vi "user1.vi"() -> ()   [LabVIEW 2017]
uses:
  people.ctl
panel:
  in  "From":T1
  in  "To":T1
  in  "Message":string
  out "error out":errorcluster
  in  "error in":errorcluster
  out "Messages":string
  in  "EXIT":bool
  in  "SEND":bool
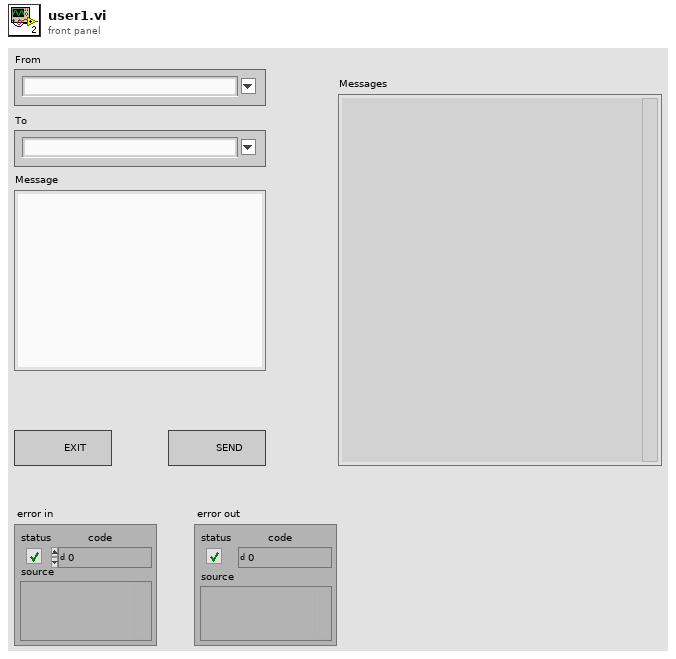
[diagram p1: front panel]
types:
  T1 = typedef "people.ctl" = string
  T2 = enum16{"open", "replace", "create", "open or create", "replace or create", "replace or create with confirmation"}
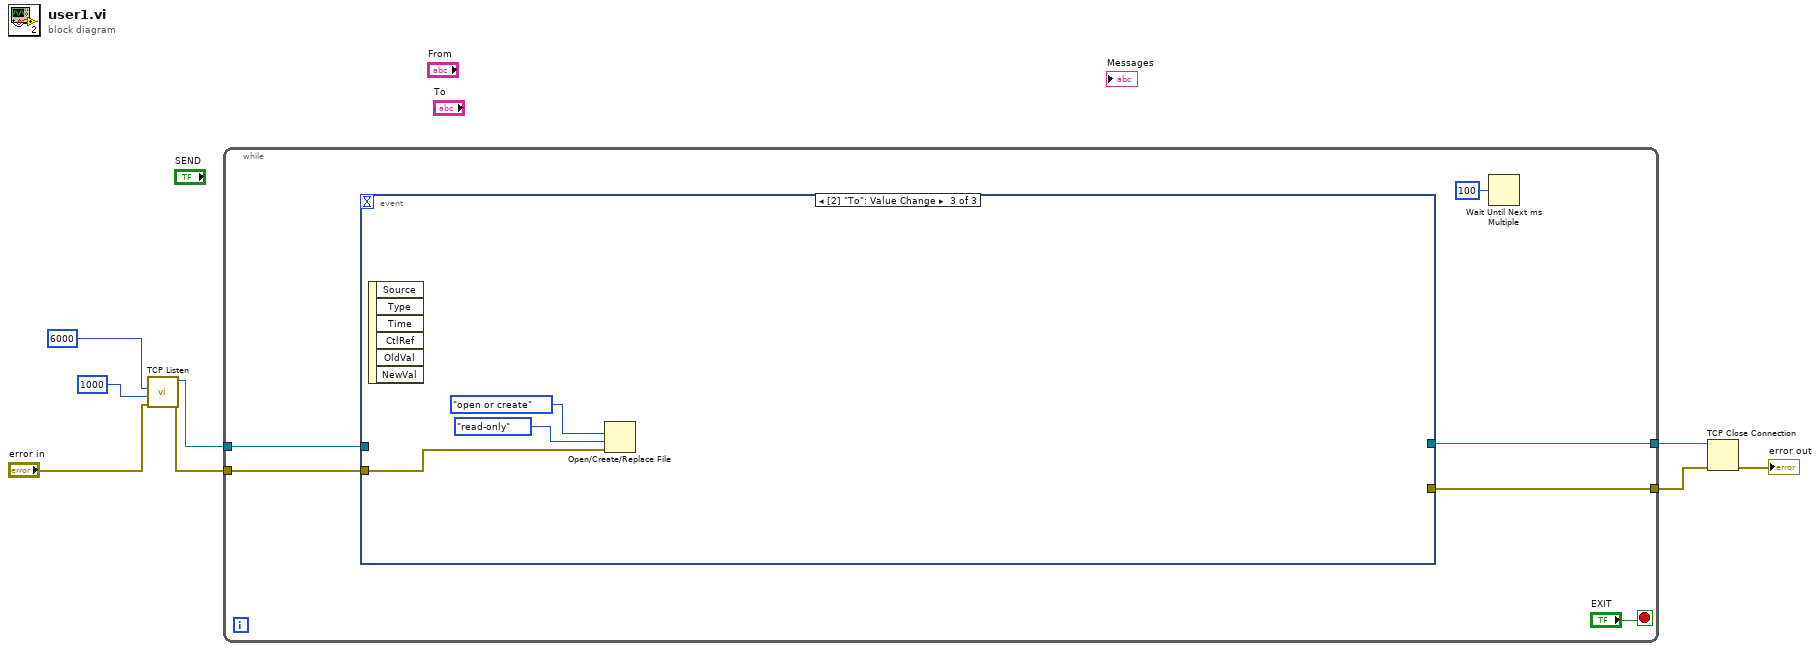
[diagram p0: block diagram]
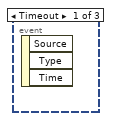
[diagram p2: hidden frame]
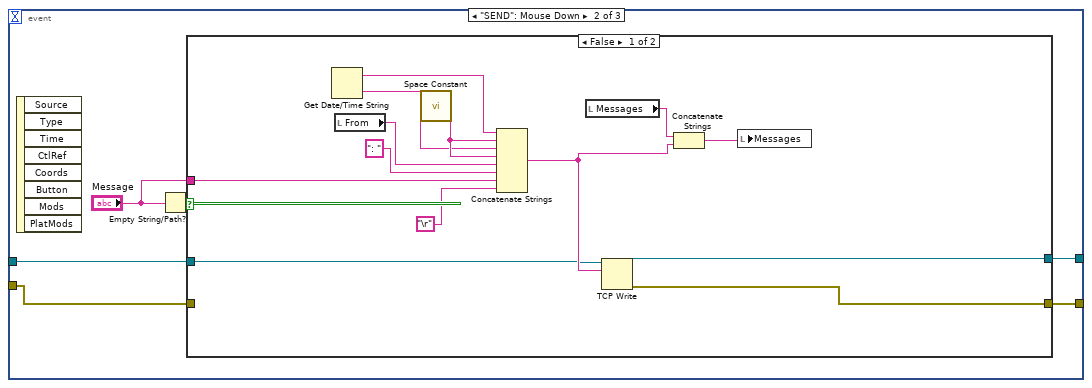
[diagram p3: hidden frame]
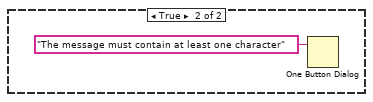
[diagram p4: hidden frame]
diagram:
  n1 = call <vilib>:"TCP Listen.vi"("error in (no error)"="error in", "timeout ms (wait forever: -1)"=1000, "port"=u16 6000 ("remote port or service name")) -> ("error out"=w2:errorcluster, "connection ID"=w3:refnum<k5>)  [unwired: 4 in, 3 out]
  n2 = while {
    tunnel: [w13] -> w8
    tunnel: [w12] -> w6
    tunnel: w3 -> [w11]
    tunnel: w2 -> [w10]
    stop <- "EXIT" stop-if-true
    n3 = event shown="[2] \"To\": Value Change" {
      selector: _ -> [_ _ _]
      dyn-events: _ -> [_ _ _]
      timeout: _ -> [_ _ _]
      tunnel: w11 -> [_ w15 _]
      tunnel: w10 -> [_ w16 w35]
      tunnel: [_ w19 _] -> w13
      tunnel: [_ w18 _] -> w12
      event Timeout {
        n4 = event-data() -> ()  [unwired: 1 in, 3 out]
      }
      event "SEND": Mouse Down {
        n5 = event-data() -> ()  [unwired: 1 in, 8 out]
        n6 = Empty String/Path?(string/path="Message") -> (empty?=w20:bool)
        n7 = case shown="False" w20 {
          tunnel: [w25 _] -> w19
          tunnel: [w24 _] -> w18
          tunnel: "Message" -> [w23 _]
          tunnel: w16 -> [_ _]
          tunnel: w15 -> [w22 _]
          frame False {
            n8 = Get Date/Time String() -> (date string=w28:string, time string=w32:string)  [unwired: 3 in]
            n9 = local read "From"() -> (w21:T1)
            n10 = call <vilib>:"Space Constant.vi"() -> ("String"=w33:string)
            n11 = Concatenate Strings(w28, w33, w32, w33, w21, ": ", w23, "\r") -> (w30:string)
            n12 = local read "Messages"() -> (w29:string)
            n13 = TCP Write(connection ID=w22, data in=w30) -> (connection ID out=w24:refnum<k5>, error out=w25:errorcluster)  [unwired: 2 in, 1 out]
            n14 = Concatenate Strings(w29, w30) -> (w31:string)
            n15 = local write "Messages"(w31) -> ()
          }
          frame True {
            n16 = One Button Dialog(message="The message must contain at least one character") -> ()  [unwired: 1 in, 1 out]
          }
        }
      }
      event Value Change {
        n17 = event-data() -> ()  [unwired: 1 in, 6 out]
        n18 = Open/Create/Replace File(error in=w35, operation (0:open)=T2."open or create", access (0:read/write)=enum16{"read/write", "read-only", "write-only"}."read-only") -> ()  [unwired: 3 in, 3 out]
      }
    }
    n19 = Wait Until Next ms Multiple(millisecond multiple=u32 100) -> ()  [unwired: 1 out]
  }
  n20 = TCP Close Connection(connection ID=w6, error in (no error)=w8) -> (error out=→"error out":errorcluster)  [unwired: 1 in, 1 out]
